vi "Get Channel List.vi"(5 "Force all(F)":bool, 11 "error in":errorcluster) -> (6 "Numb Elements":i32, 8 "Names":string[](array[string]), 10 "Ring list":cluster{"String":string, "Value":u16}[](array[cluster]), 14 "Value list":u16[](array[numeric]), 15 "error out":errorcluster)   [LabVIEW 2011]
uses:
  Channel Classification Enum.ctl
  <vilib>/Utility/VariantDataType/GetNumericInfo.vi
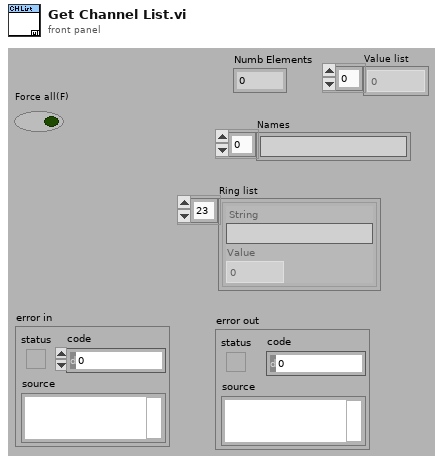
[diagram p1: front panel]
types:
  T1 = typedef "Channel Classification Enum.ctl" = enum16{"Basic", "Advanced", "Expert", "Unused"}
  T2 = enum16{"GET", "SET", "Get from Ini", "Put in Ini"}
  T3 = typedef "User Indikator.ctl" = cluster{"User Name":string, "Super User":T4}
  T4 = typedef "Super User bool indikator.ctl" = bool
  T5 = typedef "User Setting Analog Channel Bg.ctl" = cluster{"Scaling":T6, "Limits and responces":T7, "Allow Graph selection by user":bool, "Unit":u16}
  T6 = typedef "Scaling.ctl" = cluster{"Gain":dbl, "Offset":dbl}
  T7 = typedef "Alarm Setup Analog.ctl" = cluster{"Technical Error(NA)":T8, "LL":T8, "L":T8, "H":T8, "HH":T8, "Limits":T10}
  T8 = typedef "Alarm Responce.ctl" = cluster{"Action":T9, "Alarm":bool}
  T9 = typedef "Action List.ctl" = enum16{"No Action", "Stop Motor", "Turn Off HV"}
  T10 = typedef "Limits.ctl" = cluster{"LL":dbl, "L":dbl, "H":dbl, "HH":dbl}
  T11 = typedef "Fixed Analog Channel Definition.ctl" = cluster{"ID":u16, "Name":string, "Quantity":T12, "Unit":string, "Maximum upd":T13, "Comment":string, "Help file Name":string, "Help file Section ":string, "Category":T14, "User adjustable Scaling":bool, "Default Scaling":T6, "Default Unit":i32, "Classification":T1}
  T12 = typedef "Quantity enum.ctl" = enum16{"NA", "Acceleration", "Angle", "Current", "Force", "Distance", "Pressure", "Resistance", "Rotational Speed", "Speed", "Temperature", "Tension", "Torque", "Voltage", "Weight"}
  T13 = typedef "Update frequensies.ctl" = enum16{"2 Hz", "1 Hz", "0.1 Hz"}
  T14 = typedef "Channel catagory Enum.ctl" = enum16{"No Category", "Power", "Temperature", "Pressure"}
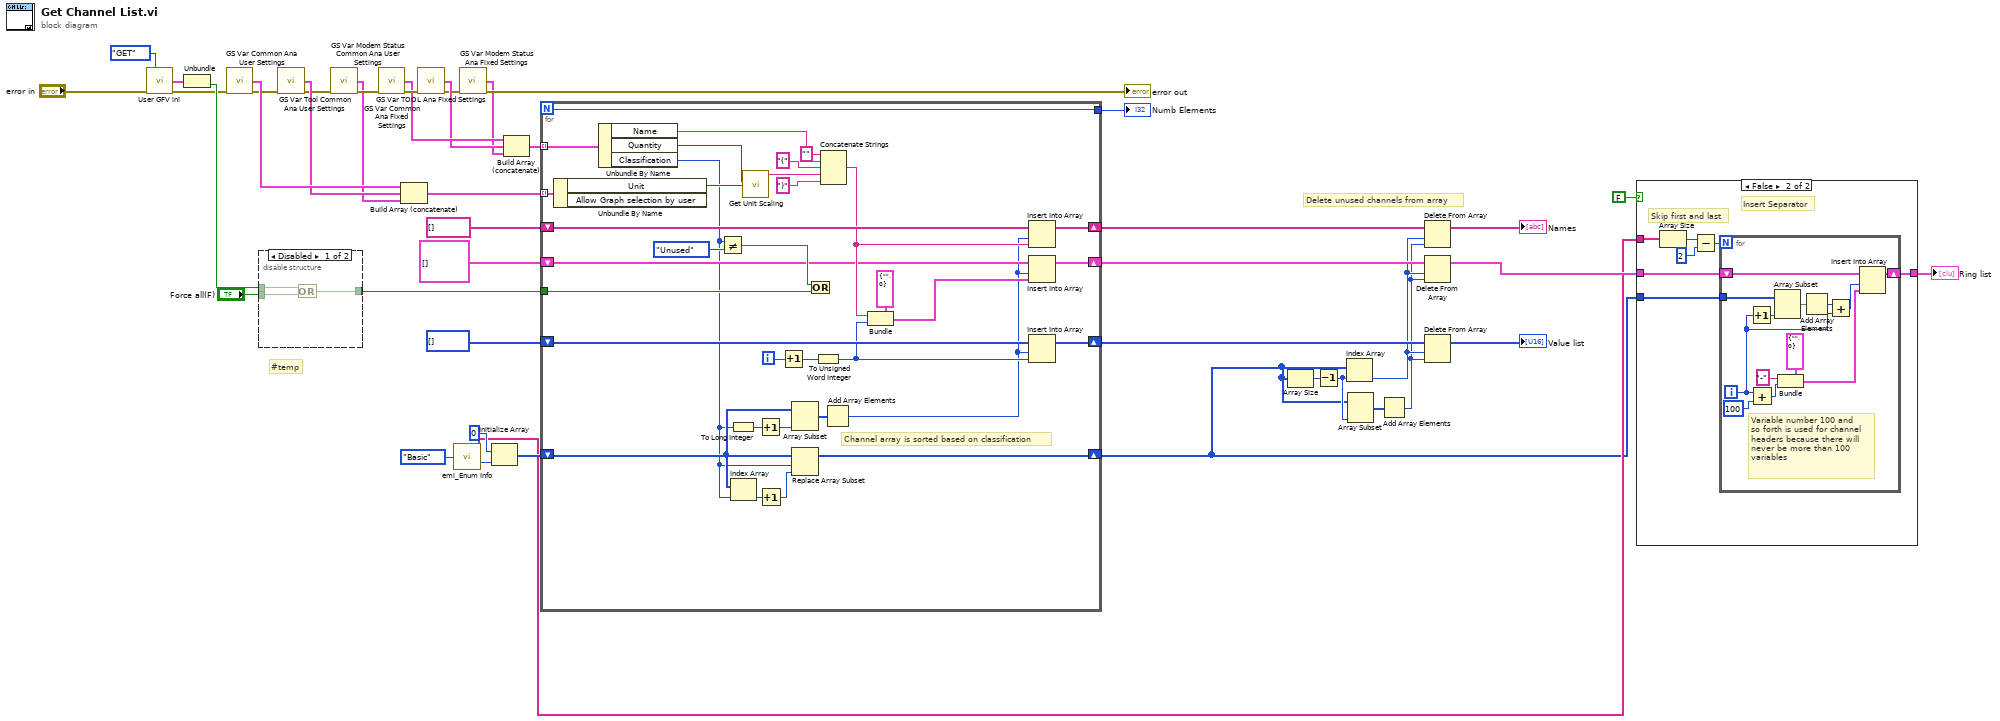
[diagram p0: block diagram]
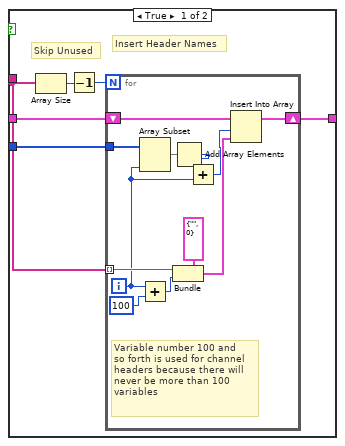
[diagram p2: hidden frame]
diagram:
  # "Delete unused channels from array"
  # "#temp"
  n1 = call "User GFV ini.vi"("Action(GET)"=T2."GET", "error in (no error)"="error in") -> ("User ID out"=w38:T3, "error out"=w31:errorcluster)  [unwired: 12 in]
  n2 = Unbundle(w38) -> ("Super User"=w34:T4)  [unwired: 1 out]
  n3 = call "GS Var Common Ana User Settings.vi"("error in (no error)"=w31) -> ("Common Analog var User set out"=w33:T5[], "error out"=w30:errorcluster)  [unwired: 12 in, 1 out]
  n4 = disable-structure shown="Disabled" {
    disable-tunnel: w34 -> [w47 _]
    disable-tunnel: [w46 w48] -> w28
    disable-tunnel: "Force all(F)" -> [w45 w48]
    frame Disabled {
      n5 = Or(x=w47, y=w45) -> (x .or. y?=w46:T4)
    }
    frame Enabled {
    }
  }
  n6 = call "GS Var Tool Common Ana User Settings.vi"("error in (no error)"=w30) -> ("Tool Analog var User settigns out"=w32:T5[], "error out"=w25:errorcluster)  [unwired: 12 in, 1 out]
  n7 = call "GS Var Modem Status Common Ana User Settings.vi"("error in (no error)"=w25) -> ("Modem Status Analog var User settigns out"=w23:T5[], "error out"=w24:errorcluster)  [unwired: 12 in, 1 out]
  n8 = call "GS Var Common Ana Fixed Settings.vi"("error in (no error)"=w24) -> ("Common Analog Var Fixed out"=w41:T11[], "error out"=w42:errorcluster)  [unwired: 12 in, 1 out]
  n9 = Build Array (concatenate)(w33, w32, w23) -> (w29:T5[])
  n10 = call "GS Var TOOL Ana Fixed Settings.vi"("error in (no error)"=w42) -> ("Tool Analog var Fixed out"=w40:T11[], "error out"=w22:errorcluster)  [unwired: 12 in, 1 out]
  n11 = call "emi_Enum Info.vi"("Enum"=Channel_Classification_Enum."Basic" ("y")) -> ("Text Elements"=w7:string[], "Numb Elements"=w18:i32)  [unwired: 11 in, 2 out]
  n12 = call "GS Var Modem Status Ana Fixed Settings.vi"("error in (no error)"=w22) -> ("Modem Status Analog var Fixed out"=w20:T11[], "error out"=→"error out":errorcluster)  [unwired: 12 in, 1 out]
  n13 = Initialize Array(0, w18) -> (w16:i32[])
  n14 = Build Array (concatenate)(w41, w40, w20) -> (w39:T11[])
  n15 = for {
    N -> [w82]
    tunnel: w39 -> [w81] mode=indexing
    tunnel: [w82] -> w43
    shift-right: [w61] -> w15
    shift-left: string[] [] -> [w72]
    shift-right: [w58] -> w14
    shift-left: cluster{"String":string, "Value":u16}[] [] -> [w60]
    tunnel: w28 -> [w74]
    tunnel: w29 -> [w73] mode=indexing
    shift-right: [w56] -> w13
    shift-left: u16[] [] -> [w57]
    shift-right: [w64] -> w1
    shift-left: w16 -> [w53]
    i -> [w79]
    # "Channel array is sorted based on classification"
    n16 = Unbundle By Name(w73) -> ("Unit"=w69:u16)  [unwired: 1 out]
    n17 = Unbundle By Name(w81) -> ("Name"=w77:string, "Quantity"=w71:T12, "Classification"=w51:T1)
    n18 = Not Equal?(x=w51, y=Channel_Classification_Enum."Unused") -> (x != y?=w67:bool)
    n19 = To Long Integer(number=w51) -> (32bit integer=w50:i32)
    n20 = Index Array(array=w53, index=w51) -> (element=w66:i32)
    n21 = call "Get Unit Scaling.vi"("Unit Index"=w69, "Quantity"=w71) -> ("Unit"=w70:string)  [unwired: 7 in, 2 out]
    n22 = Increment(x=w50) -> (x+1=w52:i32)
    n23 = Increment(x=w66) -> (x+1=w65:i32)
    n24 = Increment(x=w79) -> (x+1=w78:i32)
    n25 = Array Subset(array=w53, length=w52) -> (w63:i32[])  [unwired: 1 in]
    n26 = Replace Array Subset(array=w53, new element=w65, index=w51) -> (w64:i32[])
    n27 = Or(x=w67, y=w74) -> ()  [unwired: 1 out]
    n28 = To Unsigned Word Integer(number=w78) -> (unsigned 16bit integer=w55:u16)
    n29 = Concatenate Strings("" ("string"), w77, "(" ("string"), w70, ")" ("string")) -> (w62:string)
    n30 = Add Array Elements(numeric array=w63) -> (sum=w54:i32)
    n31 = Bundle(cluster=cluster{"String":string, "Value":u16} {"String"="", "Value"=0}, "String"=w62, "Value"=w55) -> (w59:cluster{"String":string, "Value":u16})
    n32 = Insert Into Array(array=w72, index=w54, new element=w62) -> (w61:string[])
    n33 = Insert Into Array(array=w60, index=w54, new element=w59) -> (w58:cluster{"String":string, "Value":u16}[])
    n34 = Insert Into Array(array=w57, index=w54, new element=w55) -> (w56:u16[])
  }
  "Numb Elements" <- w43
  n35 = Array Size(array=w1) -> (size(s)=w6:i32)
  n36 = Decrement(x=w6) -> (x-1=w3:i32)
  n37 = Index Array(array=w1, index=w3) -> (element=w5:i32)
  n38 = Array Subset(array=w1, length=w3) -> (w4:i32[])  [unwired: 1 in]
  n39 = Add Array Elements(numeric array=w4) -> (sum=w2:i32)
  n40 = Delete From Array(array=w15, length=w5, index=w2) -> (array with subset deleted=→"Names":string[])  [unwired: 1 out]
  n41 = Delete From Array(array=w14, length=w5, index=w2) -> (array with subset deleted=w10:cluster{"String":string, "Value":u16}[])  [unwired: 1 out]
  n42 = Delete From Array(array=w13, length=w5, index=w2) -> (array with subset deleted=→"Value list":u16[])  [unwired: 1 out]
  n43 = case shown="False" FALSE {
    tunnel: w10 -> [w88 w107]
    tunnel: w1 -> [w86 w105]
    tunnel: [w87 w106] -> w8
    tunnel: w7 -> [w83 w104]
    frame True {
      # "Insert Header Names"
      # "Skip Unused"
      n44 = Array Size(array=w83) -> (size(s)=w85:i32)
      n45 = Decrement(x=w85) -> (x-1=w84:i32)
      n46 = for {
        N: w84 -> [_]
        shift-right: [w99] -> w87
        shift-left: w88 -> [w100]
        tunnel: w83 -> [w94] mode=indexing
        tunnel: w86 -> [w92]
        i -> [w90]
        # "Variable number 100 and \nso forth is used for channel\nheaders because there will \nnever be more than 100 \nvariables"
        n47 = Array Subset(array=w92, length=w90) -> (w93:i32[])  [unwired: 1 in]
        n48 = Add(x=w90, y=100) -> (x+y=w95:i32)
        n49 = Bundle(cluster=cluster{"String":string, "Value":u16} {"String"="", "Value"=0}, "String"=w94, "Value"=w95) -> (w97:cluster{"String":string, "Value":u16})
        n50 = Add Array Elements(numeric array=w93) -> (sum=w91:i32)
        n51 = Add(x=w91, y=w90) -> (x+y=w89:i32)
        n52 = Insert Into Array(array=w100, index=w89, new element=w97) -> (w99:cluster{"String":string, "Value":u16}[])
      }
    }
    frame False {
      # "Insert Separator"
      # "Skip first and last"
      n53 = Array Size(array=w104) -> (size(s)=w103:i32)
      n54 = Subtract(x=w103, y=2) -> (x-y=w101:i32)
      n55 = for {
        N: w101 -> [_]
        shift-right: [w119] -> w106
        shift-left: w107 -> [w120]
        tunnel: w105 -> [w113]
        i -> [w111]
        # "Variable number 100 and \nso forth is used for channel\nheaders because there will \nnever be more than 100 \nvariables"
        n56 = Increment(x=w111) -> (x+1=w109:i32)
        n57 = Add(x=w111, y=100) -> (x+y=w115:i32)
        n58 = Array Subset(array=w113, length=w109) -> (w114:i32[])  [unwired: 1 in]
        n59 = Bundle(cluster=cluster{"String":string, "Value":u16} {"String"="", "Value"=0}, "String"="-", "Value"=w115) -> (w117:cluster{"String":string, "Value":u16})
        n60 = Add Array Elements(numeric array=w114) -> (sum=w112:i32)
        n61 = Add(x=w112, y=w111) -> (x+y=w110:i32)
        n62 = Insert Into Array(array=w120, index=w110, new element=w117) -> (w119:cluster{"String":string, "Value":u16}[])
      }
    }
  }
  "Ring list" <- w8
